vi "bool_change.vi"(0 "RAW":bool, 5 "bool_data_in":T1, 7 "bool_setting":T2) -> (4 "CURR":bool, 6 "bool_data_out":T1)   [LabVIEW 2019]
uses:
  TypeDef/bool_setting.ctl
  TypeDef/bool_data.ctl
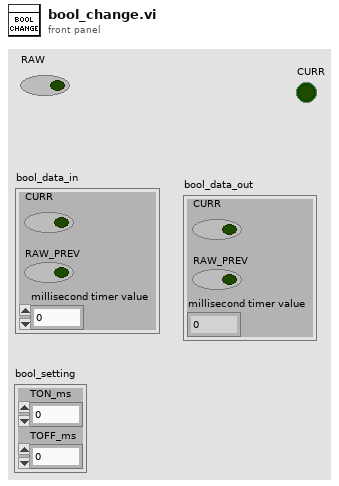
[diagram p1: front panel]
types:
  T1 = typedef "bool_data.ctl" = cluster{"CURR":bool, "RAW_PREV":bool, "millisecond timer value":u32}
  T2 = typedef "bool_setting.ctl" = cluster{"TON_ms":u32, "TOFF_ms":u32}
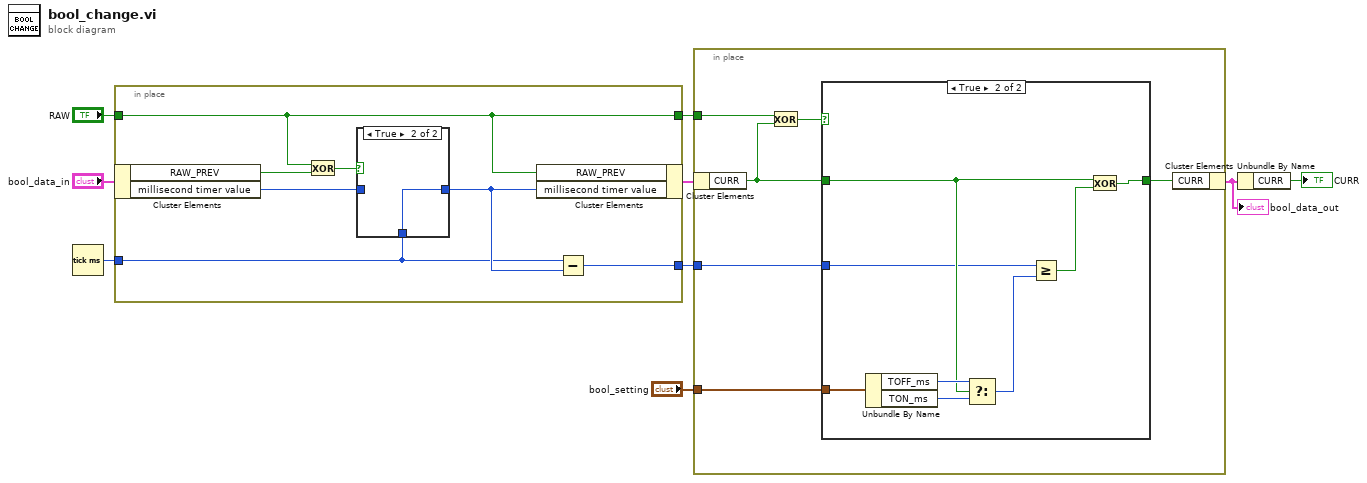
[diagram p0: block diagram]
diagram:
  n1 = Tick Count (ms)() -> (millisecond timer value=w2:u32)
  n2 = in-place {
    in-place-border: "RAW" -> [w13]
    in-place-border: [w13] -> w6
    in-place-border: w2 -> [w11]
    in-place-border: [w10] -> w1
    n3 = in-place-cluster #1("bool_data_in") -> ("RAW_PREV"=w16:bool, "millisecond timer value"=w15:u32)
    n4 = Exclusive Or(1:w16, 2:w13) -> (0:w14:bool)
    n5 = case shown="True" w14 {
      tunnel: w15 -> [w17 _]
      tunnel: [w17 w18] -> w12
      tunnel: w11 -> [_ w18]
      frame False {
      }
      frame True {
      }
    }
    n6 = in-place-cluster #1("RAW_PREV"=w13, "millisecond timer value"=w12) -> (w5:T1)
    n7 = Subtract(x=w11, y=w12) -> (x-y=w10:u32)
  }
  n8 = in-place {
    in-place-border: w6 -> [w24]
    in-place-border: "bool_setting" -> [w20]
    in-place-border: w1 -> [w19]
    n9 = in-place-cluster #2(w5) -> ("CURR"=w21:bool)
    n10 = Exclusive Or(1:w21, 2:w24) -> (0:w23:bool)
    n11 = case shown="True" w23 {
      tunnel: [w25 w33] -> w22
      tunnel: w21 -> [w25 w29]
      tunnel: w20 -> [_ w32]
      tunnel: w19 -> [_ w26]
      frame False {
      }
      frame True {
        n12 = Unbundle By Name(w32) -> ("TOFF_ms"=w31:u32, "TON_ms"=w30:u32)
        n13 = Select(t=w31, s=w29, f=w30) -> (s? t:f=w28:u32)
        n14 = Greater Or Equal?(x=w26, y=w28) -> (x >= y?=w27:bool)
        n15 = Exclusive Or(1:w27, 2:w29) -> (0:w33:bool)
      }
    }
    n16 = in-place-cluster #2("CURR"=w22) -> (w3:T1)
  }
  "bool_data_out" <- w3
  n17 = Unbundle By Name(w3) -> ("CURR"=→"CURR":bool)
